vi "COPulseProps.vi"(0 "task in":refnum<k24>, 3 "error in (no error)":errorcluster) -> (1 "DutyCycle":dbl, 4 "HighTicks":u32, 5 "HighTime":dbl, 6 "task out":refnum<k24>, 7 "LowTicks":u32, 8 "Frequency":dbl, 9 "LowTime":dbl, 10 "error out":errorcluster)   [LabVIEW 2010]
uses:
  C:/Program Files/National Instruments/LabVIEW 2010/vi.lib/ULx/ULx_LV.dll
  Program Files/National Instruments/LabVIEW 2010/vi.lib/ULx/ULx_LV.dll
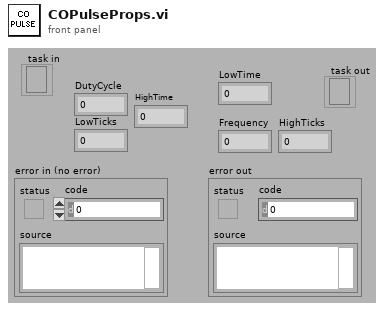
[diagram p1: front panel]
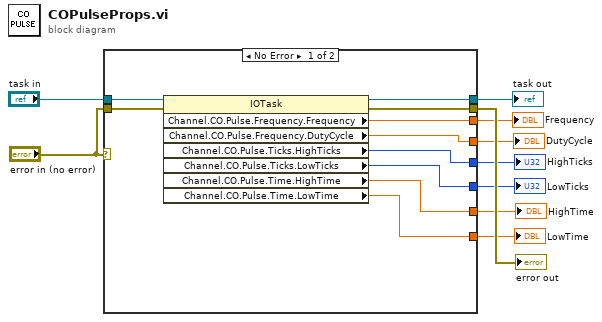
[diagram p0: block diagram]
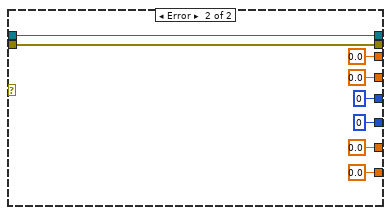
[diagram p2: hidden frame]
diagram:
  n1 = case shown="No Error" "error in (no error)" {
    tunnel: "task in" -> [w20 w28]
    tunnel: "error in (no error)" -> [w19 w27]
    tunnel: [w18 w28] -> w9
    tunnel: [w17 w27] -> w8
    tunnel: [w16 0.0 ("Channel.CO.Pulse.Frequency.Frequency")] -> w6
    tunnel: [w15 0.0 ("Channel.CO.Pulse.Frequency.DutyCycle")] -> w5
    tunnel: [w14 u32 0 ("Channel.CO.Pulse.Ticks.HighTicks")] -> w4
    tunnel: [w13 u32 0 ("Channel.CO.Pulse.Ticks.LowTicks")] -> w3
    tunnel: [w12 0.0 ("Channel.CO.Pulse.Time.HighTime")] -> w2
    tunnel: [w11 0.0 ("Channel.CO.Pulse.Time.LowTime")] -> w1
    frame No Error {
      n2 = property class="IOTask"(reference=w20, error in=w19) -> (reference out=w18:refnum<k24>, error out=w17:errorcluster, "Channel.CO.Pulse.Frequency.Frequency"=w16:dbl, "Channel.CO.Pulse.Frequency.DutyCycle"=w15:dbl, "Channel.CO.Pulse.Ticks.HighTicks"=w14:u32, "Channel.CO.Pulse.Ticks.LowTicks"=w13:u32, "Channel.CO.Pulse.Time.HighTime"=w12:dbl, "Channel.CO.Pulse.Time.LowTime"=w11:dbl)
    }
    frame Error {
    }
  }
  "task out" <- w9
  "error out" <- w8
  "Frequency" <- w6
  "DutyCycle" <- w5
  "HighTicks" <- w4
  "LowTicks" <- w3
  "HighTime" <- w2
  "LowTime" <- w1
